vi "temp chart scale adjust.vi"(0 "Control Parameters":T2={"Setpoint"=50.0, "Control bandwidth"=4.0, "Settle bandwidth"=1.0, "Integral time"=30.0, "Int\non"=TRUE, "Derivative time"=0.5, "Der\non"=TRUE, "Settle time"=60.0} {"Settle time" format="%.2f"; "Derivative time" format="%.2f"; "Integral time" format="%.2f"; "Settle bandwidth" format="%.2f"; "Control bandwidth" format="%.2f"; "Setpoint" format="%.2f"}, 7 "Scale Control In":T1, 9 "Temperature History in":refnum<vi>) -> (8 "Scale Control Out":T1, 10 "Temperature History out":refnum<vi>)   [LabVIEW 2014]
doc: "This subvi adjusts the scales on the temperature chart.\n\nPaul K Dixon\nPhysics 350\nCSUSB Physics"
uses:
  typedefs/scale control.ctl
  typedefs/control parameters.ctl
  globals/temp control global variables.vi
panel:
  # "scale adjust"
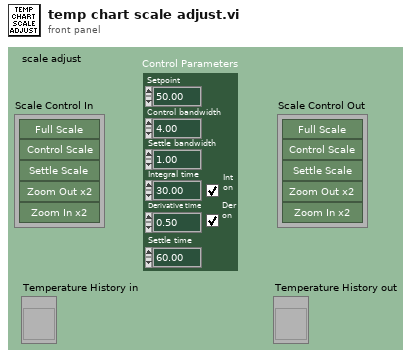
[diagram p1: front panel]
types:
  T1 = typedef "scale control.ctl" = cluster{"Full Scale":bool, "Control Scale":bool, "Settle Scale":bool, "Zoom Out":bool, "Zoom In":bool}
  T2 = typedef "control parameters.ctl" = cluster{"Setpoint":dbl, "Control bandwidth":dbl, "Settle bandwidth":dbl, "Integral time":dbl, "Int\non":bool, "Derivative time":dbl, "Der\non":bool, "Settle time":dbl}
  T3 = cluster{"temp out":dbl, dbl, dbl, dbl, dbl, dbl, dbl}[]
  T4 = cluster{"temp out":dbl, dbl, dbl, dbl, dbl, dbl, dbl}
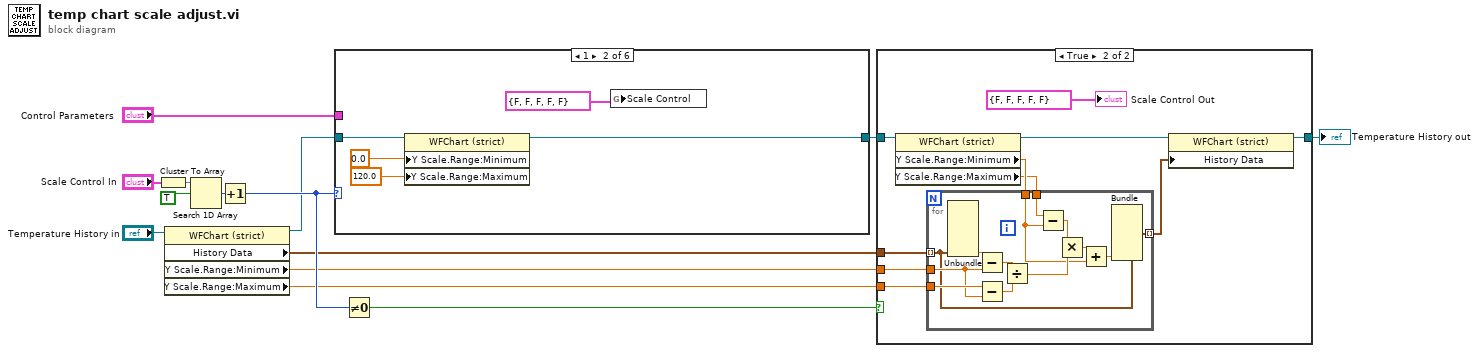
[diagram p0: block diagram]
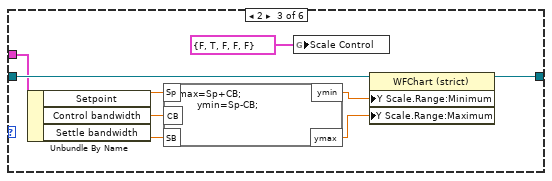
[diagram p4: hidden frame]
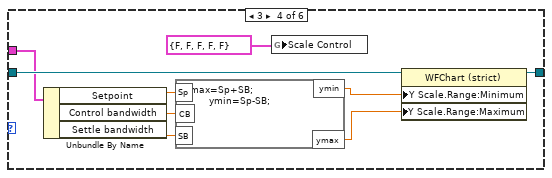
[diagram p5: hidden frame]
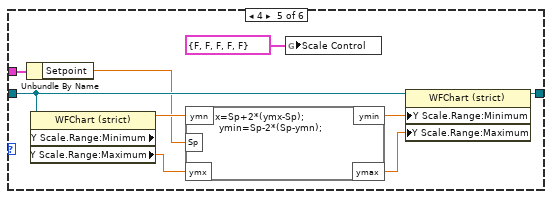
[diagram p6: hidden frame]
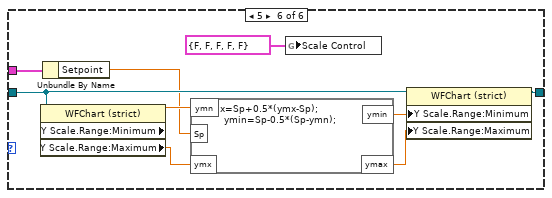
[diagram p7: hidden frame]
diagram:
  n1 = Cluster To Array(cluster="Scale Control In") -> (array=w12:bool[])
  n2 = property on="Property Node" class="WFChart (strict)"(reference="Temperature History in") -> (reference out=w9:refnum<vi>, "History Data"=w4:T3, "Y Scale.Range:Minimum"=w6:dbl, "Y Scale.Range:Maximum"=w5:dbl)  [unwired: 1 in, 1 out]
  n3 = Search 1D Array(1D array=w12, element=TRUE) -> (index of element=w14:i32)  [unwired: 1 out]
  n4 = Increment(x=w14) -> (x+1=w10:i32)
  n5 = case shown="1" w10 {
    tunnel: "Control Parameters" -> [_ _ w25 w34 w41 w50]
    tunnel: w9 -> [w15 w18 w27 w36 w43 w51]
    tunnel: [w15 w17 w26 w35 w42 w52] -> w8
    frame 0, Default {
    }
    frame 1 {
      n6 = property on="Property Node" class="WFChart (strict)"(reference=w18, "Y Scale.Range:Minimum"=0.0, "Y Scale.Range:Maximum"=120.0) -> (reference out=w17:refnum<vi>)  [unwired: 1 in, 1 out]
      n7 = global write "temp control global variables.vi" "Scale Control"(T1 {"Full Scale"=FALSE, "Control Scale"=FALSE, "Settle Scale"=FALSE, "Zoom Out"=FALSE, "Zoom In"=FALSE} ("Scale Control")) -> ()
    }
    frame 2 {
      n8 = Unbundle By Name(w25) -> ("Setpoint"=w24:dbl, "Control bandwidth"=w23:dbl, "Settle bandwidth"=w22:dbl)
      n9 = formula code="ymax=Sp+CB;\n        ymin=Sp-CB;"("Sp"=w24, "CB"=w23, "SB"=w22) -> ("ymax"=w28:dbl, "ymin"=w29:dbl)
      n10 = global write "temp control global variables.vi" "Scale Control"(T1 {"Full Scale"=FALSE, "Control Scale"=TRUE, "Settle Scale"=FALSE, "Zoom Out"=FALSE, "Zoom In"=FALSE} ("Scale Control")) -> ()
      n11 = property on="Property Node" class="WFChart (strict)"(reference=w27, "Y Scale.Range:Minimum"=w29, "Y Scale.Range:Maximum"=w28) -> (reference out=w26:refnum<vi>)  [unwired: 1 in, 1 out]
    }
    frame 3 {
      n12 = Unbundle By Name(w34) -> ("Setpoint"=w33:dbl, "Control bandwidth"=w32:dbl, "Settle bandwidth"=w31:dbl)
      n13 = formula code="ymax=Sp+SB;\n        ymin=Sp-SB;"("Sp"=w33, "CB"=w32, "SB"=w31) -> ("ymax"=w37:dbl, "ymin"=w38:dbl)
      n14 = global write "temp control global variables.vi" "Scale Control"(T1 {"Full Scale"=FALSE, "Control Scale"=FALSE, "Settle Scale"=FALSE, "Zoom Out"=FALSE, "Zoom In"=FALSE} ("Scale Control")) -> ()
      n15 = property on="Property Node" class="WFChart (strict)"(reference=w36, "Y Scale.Range:Minimum"=w38, "Y Scale.Range:Maximum"=w37) -> (reference out=w35:refnum<vi>)  [unwired: 1 in, 1 out]
    }
    frame 4 {
      n16 = Unbundle By Name(w41) -> ("Setpoint"=w40:dbl)
      n17 = property on="Property Node" class="WFChart (strict)"(reference=w43) -> ("Y Scale.Range:Minimum"=w45:dbl, "Y Scale.Range:Maximum"=w44:dbl)  [unwired: 1 in, 2 out]
      n18 = formula code="ymax=Sp+2*(ymx-Sp);\n        ymin=Sp-2*(Sp-ymn);"("ymn"=w45, "Sp"=w40, "ymx"=w44) -> ("ymax"=w46:dbl, "ymin"=w47:dbl)
      n19 = global write "temp control global variables.vi" "Scale Control"(T1 {"Full Scale"=FALSE, "Control Scale"=FALSE, "Settle Scale"=FALSE, "Zoom Out"=FALSE, "Zoom In"=FALSE} ("Scale Control")) -> ()
      n20 = property on="Property Node" class="WFChart (strict)"(reference=w43, "Y Scale.Range:Minimum"=w47, "Y Scale.Range:Maximum"=w46) -> (reference out=w42:refnum<vi>)  [unwired: 1 in, 1 out]
    }
    frame 5 {
      n21 = property on="Property Node" class="WFChart (strict)"(reference=w51) -> ("Y Scale.Range:Minimum"=w54:dbl, "Y Scale.Range:Maximum"=w53:dbl)  [unwired: 1 in, 2 out]
      n22 = Unbundle By Name(w50) -> ("Setpoint"=w49:dbl)
      n23 = formula code="ymax=Sp+0.5*(ymx-Sp);\n        ymin=Sp-0.5*(Sp-ymn);"("ymn"=w54, "Sp"=w49, "ymx"=w53) -> ("ymax"=w55:dbl, "ymin"=w56:dbl)
      n24 = global write "temp control global variables.vi" "Scale Control"(T1 {"Full Scale"=FALSE, "Control Scale"=FALSE, "Settle Scale"=FALSE, "Zoom Out"=FALSE, "Zoom In"=FALSE} ("Scale Control")) -> ()
      n25 = property on="Property Node" class="WFChart (strict)"(reference=w51, "Y Scale.Range:Minimum"=w56, "Y Scale.Range:Maximum"=w55) -> (reference out=w52:refnum<vi>)  [unwired: 1 in, 1 out]
    }
  }
  n26 = Not Equal To 0?(x=w10) -> (x != 0?=w7:bool)
  n27 = case shown="True" w7 {
    tunnel: w8 -> [w57 w67]
    tunnel: w4 -> [_ w65]
    tunnel: w6 -> [_ w64]
    tunnel: w5 -> [_ w63]
    tunnel: [w57 w59] -> w2
    frame False {
    }
    frame True {
      n28 = property on="Property Node" class="WFChart (strict)"(reference=w67) -> (reference out=w66:refnum<vi>, "Y Scale.Range:Minimum"=w62:dbl, "Y Scale.Range:Maximum"=w61:dbl)  [unwired: 1 in, 1 out]
      n29 = for {
        tunnel: w65 -> [w70] mode=indexing
        tunnel: w64 -> [w78]
        tunnel: w63 -> [w79]
        tunnel: w62 -> [w72]
        tunnel: w61 -> [w75]
        tunnel: [w68] -> w60 mode=indexing
        n30 = Unbundle(w70) -> (w80:dbl)  [unwired: 6 out]
        n31 = Subtract(x=w80, y=w78) -> (x-y=w77:dbl)
        n32 = Subtract(x=w79, y=w78) -> (x-y=w76:dbl)
        n33 = Divide(x=w77, y=w76) -> (x/y=w73:dbl)
        n34 = Subtract(x=w75, y=w72) -> (x-y=w74:dbl)
        n35 = Multiply(x=w74, y=w73) -> (x*y=w71:dbl)
        n36 = Add(x=w71, y=w72) -> (x+y=w69:dbl)
        n37 = Bundle(cluster=w70, w69) -> (w68:T4)  [unwired: 6 out]
      }
      n38 = property on="Property Node" class="WFChart (strict)"(reference=w66, "History Data"=w60) -> (reference out=w59:refnum<vi>)  [unwired: 1 in, 1 out]
      "Scale Control Out" <- T1 {"Full Scale"=FALSE, "Control Scale"=FALSE, "Settle Scale"=FALSE, "Zoom Out"=FALSE, "Zoom In"=FALSE} ("Scale Control")
    }
  }
  "Temperature History out" <- w2
